vi "Pre Launch Init.vi"(11 "Instr Actor in":refnum<class "Instr Actor.lvclass">) -> (0 "error out":errorcluster, 3 "Instr Actor out":refnum<class "Instr Actor.lvclass">)   [LabVIEW 2014, in "Instrument Library.lvlib" / "Instr Actor.lvclass"]
doc: "(<B>Filename</B>: Actor Framework.lvlib:Actor.lvclass:Pre Launch Init.vi)\n\nDefines behavior that occurs after the Launch Nested Actor method is invoked but before the actor's Actor Core method begins running.\n\nBy default, this method does nothing. A descendant class may override it to define behavior."
uses:
  Instr Actor.lvclass
  reusable/Command/Command.lvclass
  reusable/Data/Data.lvclass
  reusable/Session APIs/File Access/Config Data/Config Data.lvclass
  reusable/Session APIs/Session Log/System Log.lvclass
  reusable/Session APIs/Session Log/System Log.lvclass/System Log.ctl
  reusable/Session APIs/File Access/Config Data/Config Data.lvclass/Config Data.ctl
  Instr Actor.lvclass/Instr Actor.ctl
  reusable/Instrument/Instrument.lvclass/Instrument.ctl
  reusable/Instrument/state.ctl
  reusable/Instrument/Write Log Session.vi
  reusable/Instrument/Write Data Notifier.vi
  reusable/Instrument/Write CMD.vi
  reusable/Instrument/Write Cfg Session.vi
  reusable/Session APIs/Session Log/Accessors/Write Main Path.vi
  reusable/Session APIs/File Access/Config Data/Accessors/Write Cfg Path.vi
  Controller/xGlobal Data.vi
  SuperActor/Ex Nested.lvclass
  reusable/Instrument/Instrument.lvclass
  <userlib>/_Session Fwk/Session - Root.lvclass
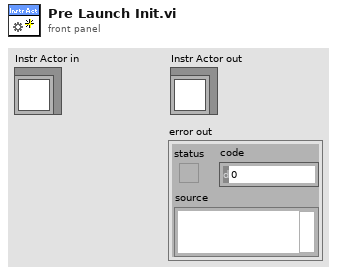
[diagram p1: front panel]
types:
  T1 = typedef "Session - Root.lvclass/Session Handle.ctl" = refnum<data-value>
  T2 = typedef "Instrument.lvclass/state.ctl" = enum8{"Configure", "Acquire", "Wait", "Quit", "Handle Error", "NOOP"}
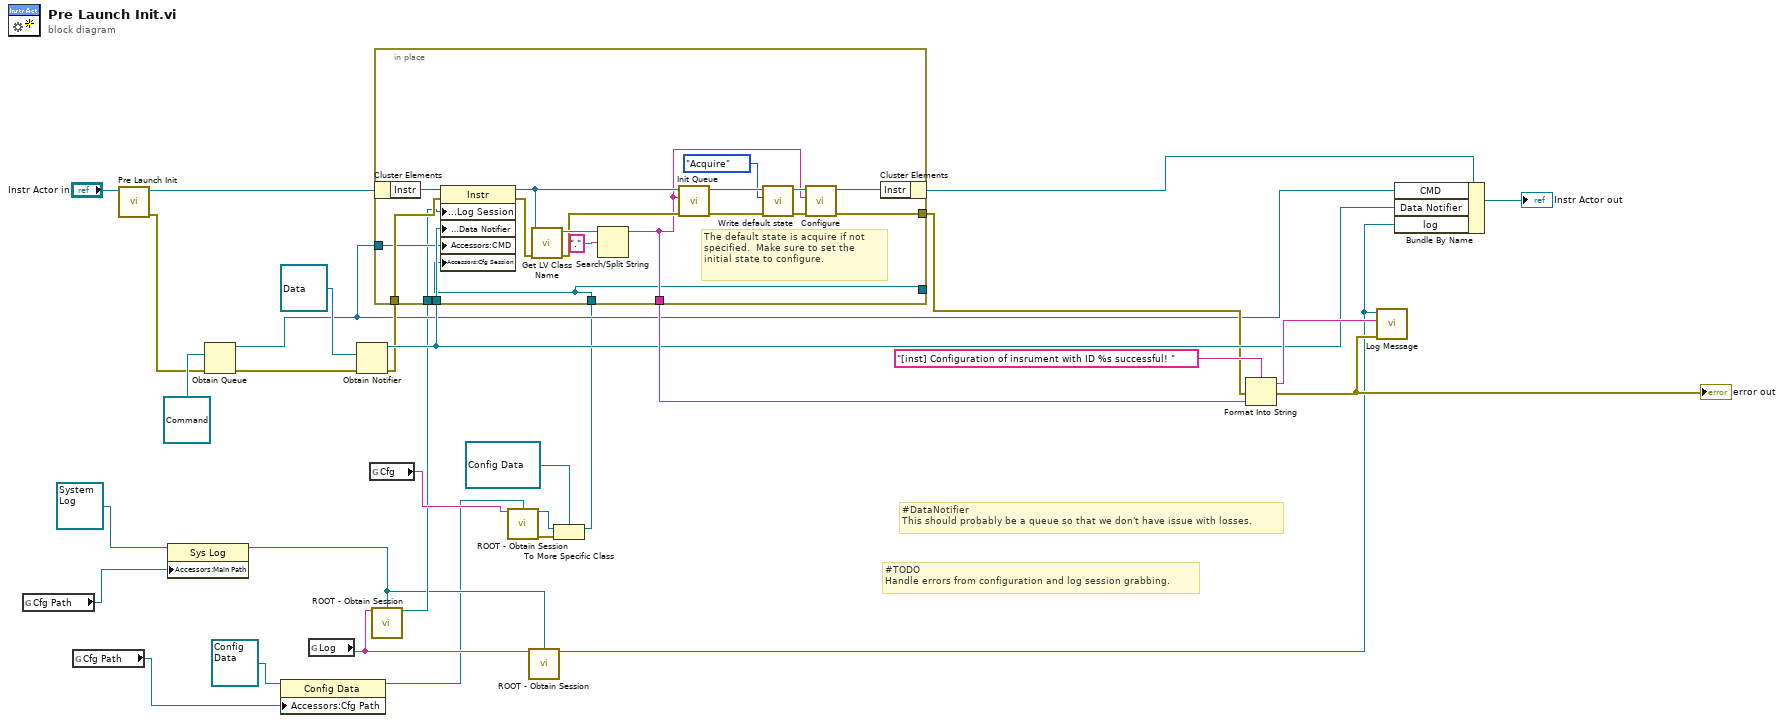
[diagram p0: block diagram]
diagram:
  # "#TODO\nHandle errors from configuration and log session grabbing."
  # "#DataNotifier\nThis should probably be a queue so that we don't have issue with losses."
  n1 = global read "xGlobal Data.vi" "Cfg Path"() -> (w8:path)
  n2 = global read "xGlobal Data.vi" "Cfg Path"() -> (w2:path)
  n3 = call-parent "Pre Launch Init.vi"("Actor in"="Instr Actor in") -> ("error out"=w17:errorcluster, "Actor out"=w26:refnum<class "Instr Actor.lvclass">)  [unwired: 9 in]
  n4 = property class="Sys Log"(reference=refnum<class "System Log.lvclass"> refnum ("Sys Log"), "Accessors:Main Path"=w8) -> (reference out=w7:refnum<class "System Log.lvclass">)  [unwired: 1 in, 1 out]
  n5 = Obtain Queue(element data type=refnum<class "Command.lvclass"> refnum ("CMD"), error in (no error)=w17) -> (queue out=w15:refnum<queue>, error out=w16:errorcluster)  [unwired: 3 in, 1 out]
  n6 = property class="Config Data"(reference=refnum<class "Config Data.lvclass"> refnum ("Config Data"), "Accessors:Cfg Path"=w2) -> (reference out=w1:refnum<class "Config Data.lvclass">)  [unwired: 1 in, 1 out]
  n7 = global read "xGlobal Data.vi" "Log"() -> (w6:string)
  n8 = Obtain Notifier(notification data type=refnum<class "Data.lvclass"> refnum ("Base Data Lib:Data"), error in (no error)=w16) -> (notifier out=w21:refnum<notifier>, error out=w20:errorcluster)  [unwired: 2 in, 1 out]
  n9 = global read "xGlobal Data.vi" "Cfg"() -> (w11:string)
  n10 = call <userlib>:"ROOT - Obtain Session.vi"("Session Name ()"=w6, "OBJ - Session"=w7) -> ("Session Handle"=w10:T1)  [unwired: 11 in, 2 out]
  n11 = call <userlib>:"ROOT - Obtain Session.vi"("Session Name ()"=w11, "OBJ - Session"=w1) -> ("Session Handle"=w12:T1, "error out"=w13:errorcluster)  [unwired: 11 in, 1 out]
  n12 = call <userlib>:"ROOT - Obtain Session.vi"("Session Name ()"=w6, "OBJ - Session"=w7) -> ("Session Handle"=w5:T1)  [unwired: 11 in, 2 out]
  n13 = To More Specific Class(target class=refnum<data-value> refnum ("Session Handle"), reference=w12, error in=w13) -> (specific class reference=w4:refnum<data-value>)  [unwired: 1 out]
  n14 = in-place {
    in-place-border: [w43] -> w18
    in-place-border: [w36] -> w25
    in-place-border: w21 -> [w35]
    in-place-border: w20 -> [w34]
    in-place-border: w15 -> [w33]
    in-place-border: w10 -> [w32]
    in-place-border: w4 -> [w31]
    in-place-border: [w31] -> _
    # "The default state is acquire if not specified.  Make sure to set the initial state to configure."
    n15 = in-place-cluster #1(w26) -> ("Instr"=w39:refnum<class "Instrument.lvclass">)
    n16 = property class="Instr"(reference=w39, error in=w34, "Accessors:Log Session"=w32, "Accessors:Data Notifier"=w35, "Accessors:CMD"=w33, "Accessors:Cfg Session"=w31) -> (reference out=w38:refnum<class "Instrument.lvclass">, error out=w37:errorcluster)
    n17 = call <vilib>:"Get LV Class Name.vi"("error in (no error)"=w37, "object"=w38) -> ("error out"=w40:errorcluster, "class name"=w41:string)  [unwired: 8 in]
    n18 = Search/Split String(string=w41, search string/char (-)="." ("regular expression")) -> (substring before match=w36:string)  [unwired: 1 in, 2 out]
    n19 = call "Init Queue.vi"("error in"=w40, "queue_name"=w36, "Instrument in"=w38) -> ("error out"=w48:errorcluster, "Instrument out"=w49:refnum<class "Instrument.lvclass">)  [unwired: 7 in]
    n20 = call "Write default state.vi"("error in (no error)"=w48, "instr state"=state."Acquire", "Instrument in"=w49) -> ("error out"=w45:errorcluster, "Instrument out"=w46:refnum<class "Instrument.lvclass">)  [unwired: 7 in]
    n21 = call-dynamic "Configure.vi"("error in"=w45, "name"=w36, "Instrument in"=w46) -> ("error out"=w43:errorcluster, "Instrument out"=w44:refnum<class "Instrument.lvclass">)  [unwired: 7 in]
    n22 = in-place-cluster #1("Instr"=w44) -> (w29:refnum<class "Instr Actor.lvclass">)
  }
  n23 = Format Into String(format string="[inst] Configuration of insrument with ID %s successful! " ("MSG In"), error in=w18, w25) -> (resulting string=w23:string, error out=w19:errorcluster)  [unwired: 1 in]
  "error out" <- w19
  n24 = call "Log Message.vi"("error in"=w19, "MSG In"=w23, "session in"=w5) -> ()  [unwired: 7 in, 2 out]
  n25 = Bundle By Name(cluster=w29, "CMD"=w15, "Data Notifier"=w21, "log"=w5) -> (→"Instr Actor out":refnum<class "Instr Actor.lvclass">)
